vi "Modules - StartUp.vi"(8 "Error In":errorcluster, 11 "List of Modules":string[](array[string])) -> (0 "Error Out":errorcluster, 3 "Module Ref":refnum<vi>[](array[refnum]), 4 "Force Exit":bool)   [LabVIEW 2019]
uses:
  Controls/StartUp - States.ctl
  Controls/FGV States.ctl
  <vilib>/Utility/error.llb/DialogType.ctl
panel:
  out "Version":string
  out "Stop":bool
  out "Status":string
  # "System Initializing...."
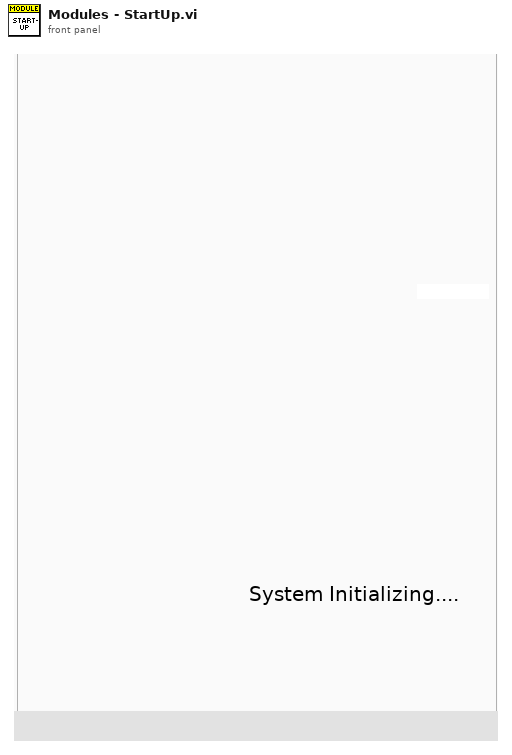
[diagram p1: front panel]
types:
  T1 = typedef "StartUp - States.ctl" = enum16{"Init Variables", "Load Configuration", "Load Modules", "Check Video", "Close"}
  T2 = typedef "FGV States.ctl" = enum16{"Read", "Write"}
  T3 = enum32{"invalid app kind", "Development System", "Run Time System", "Student Edition", "Embedded LabVIEW", "Evaluation", "Custom"}
  T4 = cluster{"Station Name":string, "Key Value":string[], "Key Names":string[]}[]
  T5 = typedef "DialogType.ctl" = u16
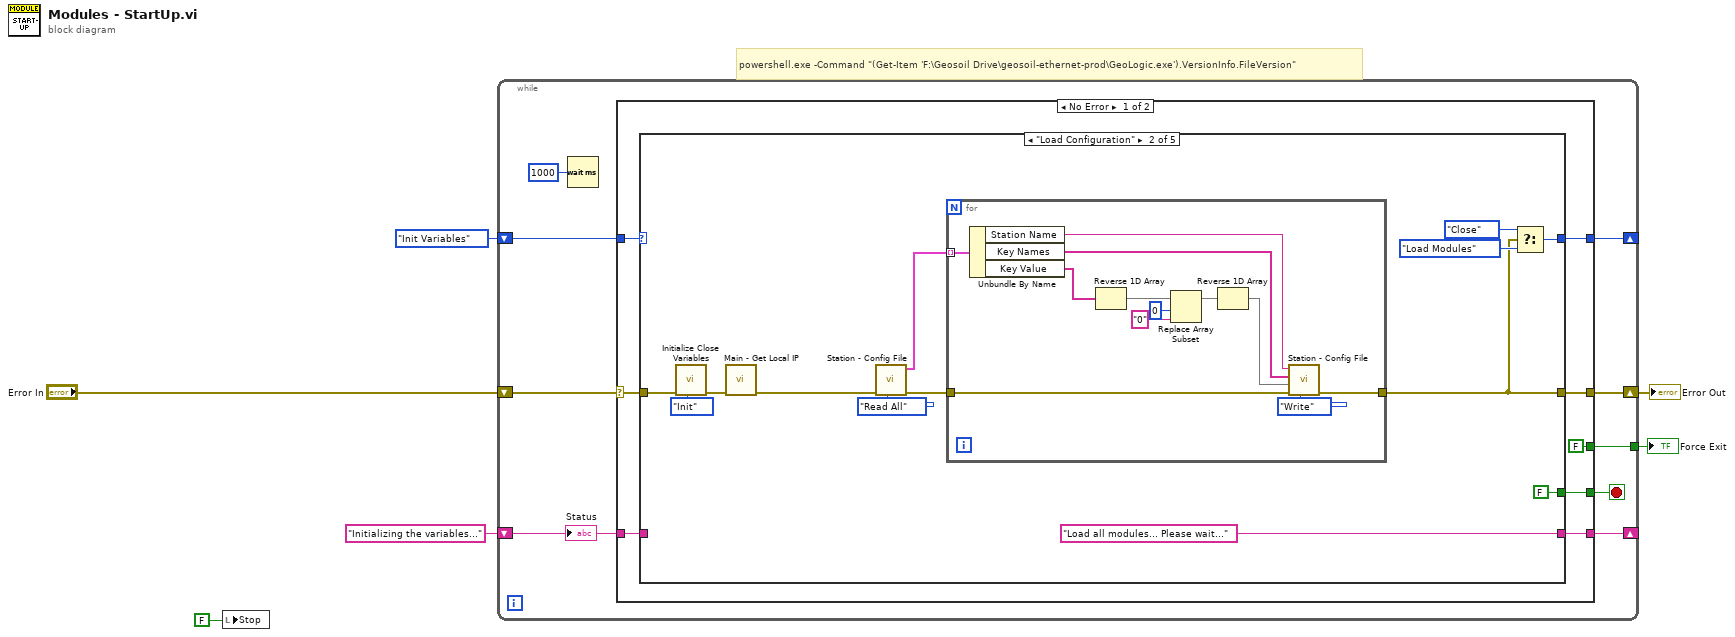
[diagram p0: block diagram]
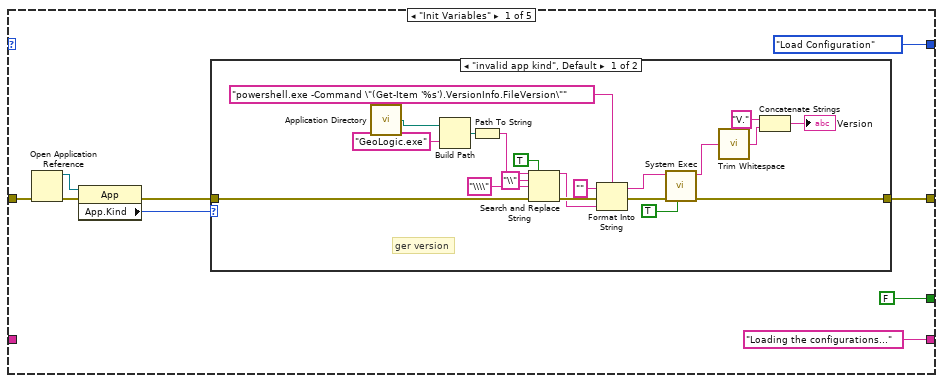
[diagram p2: hidden frame]
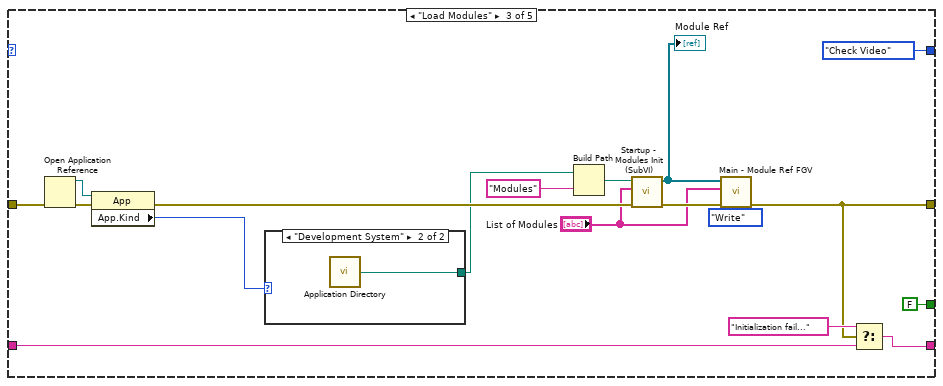
[diagram p4: hidden frame]
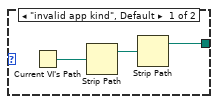
[diagram p5: hidden frame]
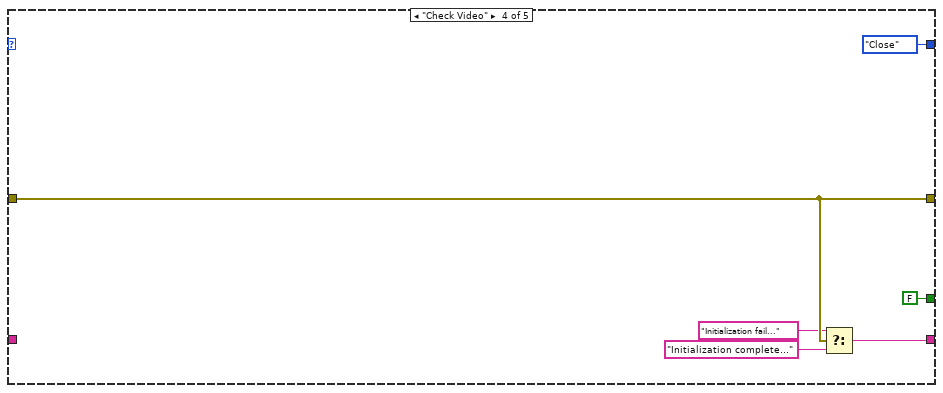
[diagram p6: hidden frame]
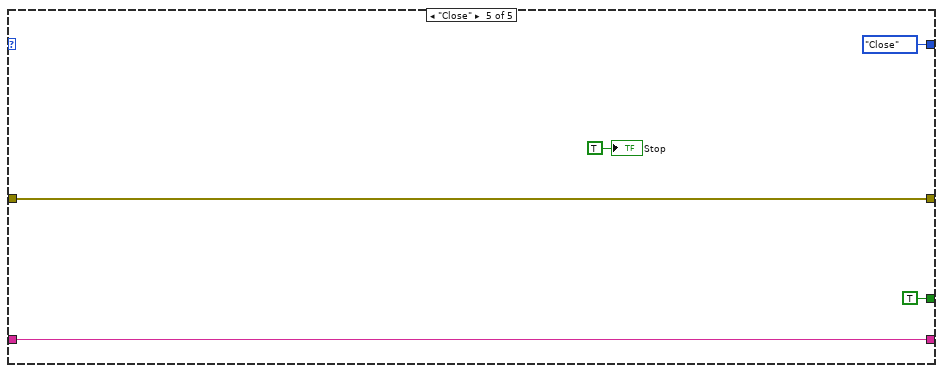
[diagram p7: hidden frame]
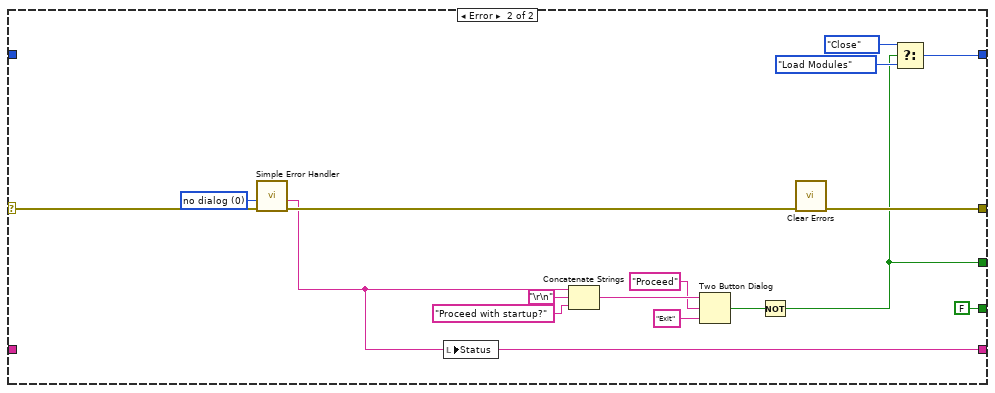
[diagram p8: hidden frame]
diagram:
  # "powershell.exe -Command \"(Get-Item 'F:\\Geosoil Drive\\geosoil-ethernet-prod\\GeoLogic.exe').VersionInfo.FileVersion\""
  n1 = local write "Stop"(FALSE ("Video Done")) -> ()
  n2 = while {
    shift-right: [w13] -> _
    shift-left: StartUp_-_States."Init Variables" -> [w14]
    shift-right: [w10] -> _
    shift-left: "Initializing the variables..." -> [w11]
    tunnel: [w9] -> w4
    shift-right: [w7] -> w3
    shift-left: "Error In" -> [w8]
    stop <- w15 stop-if-true
    n3 = Wait (ms)(milliseconds to wait=u32 1000) -> ()  [unwired: 1 out]
    n4 = case shown="No Error" w8 {
      selector: w8 -> [w16 w127]
      tunnel: [w22 FALSE] -> w15
      tunnel: [w20 w124] -> w7
      tunnel: w14 -> [w23 _]
      tunnel: [w21 w117] -> w13
      tunnel: w11 -> [w19 _]
      tunnel: [w18 w114] -> w10
      tunnel: [FALSE w115] -> w9
      frame No Error {
        n5 = case shown="\"Load Configuration\"" w23 {
          tunnel: [FALSE FALSE FALSE FALSE TRUE] -> w22
          tunnel: [StartUp_-_States."Load Configuration" w63 StartUp_-_States."Check Video" StartUp_-_States."Close" StartUp_-_States."Close"] -> w21
          tunnel: [w29 w56 w81 w105 w108] -> w20
          tunnel: w19 -> [_ _ w83 _ w109]
          tunnel: ["Loading the configurations..." "Load all modules... Please wait..." ("Status") w82 w102 w109] -> w18
          tunnel: w16 -> [w25 w61 w88 w105 w108]
          frame "Init Variables" {
            n6 = Open Application Reference(8:w25) -> (0:w28:errorcluster, 3:w27:refnum<vi>)  [unwired: 3 in]
            n7 = property class="App"(reference=w27, error in=w28) -> (error out=w26:errorcluster, "App.Kind"=w24:T3)  [unwired: 1 out]
            n8 = case shown="\"invalid app kind\", Default" w24 {
              tunnel: [w37 w53] -> w29
              tunnel: w26 -> [w34 w53]
              frame "invalid app kind", Default {
                # "ger version"
                n9 = call <vilib>:"Application Directory.vi"() -> ("Application Directory"=w52:path)
                n10 = Build Path(base path=w52, name or relative path="GeoLogic.exe") -> (appended path=w50:path)
                n11 = Path To String(path=w50) -> (string=w49:string)
                n12 = Search and Replace String(replace all?=TRUE ("replace all? (F)"), input string=w49, search string="\\", replace string="\\\\" ("replace string (\"\")"), error in=w34) -> (result string=w43:string, error out=w45:errorcluster)  [unwired: 3 in, 2 out]
                n13 = Format Into String(format string="powershell.exe -Command \"(Get-Item '%s').VersionInfo.FileVersion\"" ("name or relative path"), initial string="", error in=w45, w43) -> (resulting string=w36:string, error out=w38:errorcluster)
                n14 = call <vilib>:"System Exec.vi"("run minimized? (F)"=TRUE, "error in (no error)"=w38, "command line"=w36) -> ("error out"=w37:errorcluster, "standard output"=w33:string)  [unwired: 5 in, 2 out]
                n15 = call <vilib>:"Trim Whitespace.vi"("string"=w33) -> ("trimmed string"=w40:string)  [unwired: 1 in]
                n16 = Concatenate Strings("V." ("string"), w40) -> (→"Version":string)
              }
              frame "Development System" {
              }
            }
          }
          frame "Load Configuration" {
            n17 = call "Initialize Close Variables.vi"("Action"=enum16{"Init", "Close"}."Init", "error in (no error)"=w61) -> ("error out"=w55:errorcluster)  [unwired: 9 in]
            n18 = call "Main - Get Local IP.vi"("error in"=w55) -> ("error out"=w54:errorcluster)  [unwired: 10 in]
            n19 = call "Station - Config File.vi"("Action"=enum16{"Write", "Read", "Read All", "Remove"}."Read All", "error in (no error)"=w54) -> ("error out"=w57:errorcluster, "Value Out"=w58:T4)  [unwired: 8 in]
            n20 = for {
              tunnel: w58 -> [w78] mode=indexing
              tunnel: w57 -> [w71]
              tunnel: [w72] -> w56
              n21 = Unbundle By Name(w78) -> ("Station Name"=w70:string, "Key Names"=w69:string[], "Key Value"=w75:string[])
              n22 = Reverse 1D Array(array=w75) -> (reversed array=w67:string[])
              n23 = Replace Array Subset(array=w67, new element="0" ("new element/subarray"), index=0) -> (w73:string[])
              n24 = Reverse 1D Array(array=w73) -> (reversed array=w68:string[])
              n25 = call "Station - Config File.vi"("Action"=enum16{"Write", "Read", "Read All", "Remove"}."Write", "error in (no error)"=w71, "Value"=w68, "Key Name"=w69, "Station Name"=w70) -> ("error out"=w72:errorcluster)  [unwired: 5 in, 1 out]
            }
            n26 = Select(t=StartUp_-_States."Close", s=w56, f=StartUp_-_States."Load Modules") -> (s? t:f=w63:T1)
          }
          frame "Load Modules" {
            n27 = Open Application Reference(8:w88) -> (0:w92:errorcluster, 3:w91:refnum<vi>)  [unwired: 3 in]
            n28 = property class="App"(reference=w91, error in=w92) -> (error out=w87:errorcluster, "App.Kind"=w86:T3)  [unwired: 1 out]
            n29 = case shown="\"Development System\"" w86 {
              tunnel: [w97 w100] -> w85
              frame "invalid app kind", Default {
                n30 = Current VI's Path() -> (path=w99:path)
                n31 = Strip Path(path=w99) -> (stripped path=w98:path)  [unwired: 1 out]
                n32 = Strip Path(path=w98) -> (stripped path=w97:path)  [unwired: 1 out]
              }
              frame "Development System" {
                n33 = call <vilib>:"Application Directory.vi"() -> ("Application Directory"=w100:path)
              }
            }
            n34 = Build Path(base path=w85, name or relative path="Modules") -> (appended path=w90:path)
            n35 = call "Startup - Modules Init (SubVI).vi"("Error In"=w87, "VIs name"="List of Modules", "Path to Modules Folder"=w90) -> ("Error Out"=w94:errorcluster, "Module Refnum"=w80:refnum<vi>[])  [unwired: 7 in]
            "Module Ref" <- w80
            n36 = call "Main - Module Ref FGV.vi"("Action"=FGV_States."Write", "error In"=w94, "Module Name"="List of Modules", "Module Ref In"=w80) -> ("error out"=w81:errorcluster)  [unwired: 5 in, 2 out]
            n37 = Select(t="Initialization fail...", s=w81, f=w83) -> (s? t:f=w82:string)
          }
          frame "Check Video" {
            n38 = Select(t="Initialization fail...", s=w105, f="Initialization complete...") -> (s? t:f=w102:string)
          }
          frame "Close" {
            "Stop" <- TRUE ("Stop")
          }
        }
      }
      frame Error {
        w125 = T5 0 items=["no dialog", "OK message", "continue or stop message", "OK message + warnings", "continue/stop + warnings"] ("type of dialog (OK msg:1)")
        n39 = call <vilib>:"Simple Error Handler.vi"("type of dialog (OK msg:1)"=w125, "error in (no error)"=w127) -> ("source out"=w114:string, "error out"=w126:errorcluster)  [unwired: 3 in, 3 out]
        n40 = local write "Status"(w114) -> ()
        n41 = Concatenate Strings(w114, "\r\n", "Proceed with startup?" ("string")) -> (w121:string)
        n42 = Two Button Dialog(message=w121, 1:"Exit" ("string"), 2:"Proceed" ("string")) -> (T button?=w116:bool)
        n43 = Not(x=w116) -> (.not. x?=w115:bool)
        n44 = call <vilib>:"Clear Errors.vi"("error in (no error)"=w126) -> ("error out"=w124:errorcluster)  [unwired: 5 in, 1 out]
        n45 = Select(t=StartUp_-_States."Close", s=w115, f=StartUp_-_States."Load Modules") -> (s? t:f=w117:T1)
      }
    }
    "Status" <- w11
  }
  "Error Out" <- w3
  "Force Exit" <- w4
